vi "gatherdata_bakup2.vi"() -> ()   [LabVIEW 2011]
uses:
  <vilib>/FPGAPlugInAG/sbRIO-9606/niLvFpga_Open_sbRIO-9606.vi
  <vilib>/rvi/interface/common/dynamic/niFpgaDynamicAddResources.vi
  <vilib>/Utility/error.llb/Error Cluster From Error Code.vi
  <vilib>/rvi/errors/niLvFpgaAdjustHostInterfaceError.vi
  <vilib>/rvi/interface/nirviOpenFPGA/nirviOpenFPGA.xnode
  labview/FPGA Bitfiles/natcar_FPGATarget_Top-Level_610FB000.lvbitx
  <vilib>/rvi/interface/nirviReadWriteControl/nirviReadWriteControl.xnode
  NiFpgaLv.dll
  <vilib>/rvi/interface/Simulation/niFpgaSimulationCallBeginRW.vi
panel:
  in  "stop":bool
  in  "Save Path and Filename":path
  out "AI7":u16
  out "AI6":u16
  out "AI5":u16
  out "AI4":u16
  out "AI3":u16
  out "AI2":u16
  out "AI1":u16
  out "AI0":u16
  in  "#pts to avg":dbl=100000.0
  out "Waiting":bool
  out "Saving\nData":bool
  out "Getting\nData":bool
  in  "distance":dbl
  in  "Record":bool
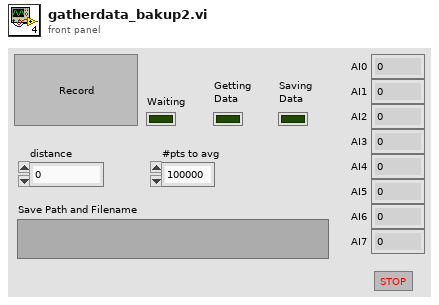
[diagram p1: front panel]
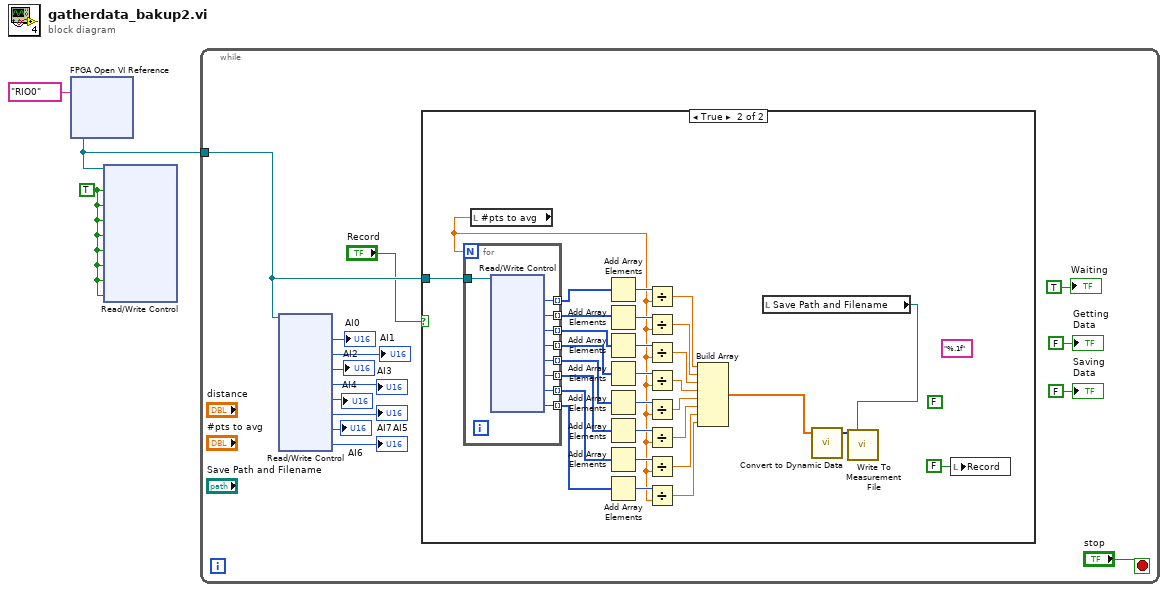
[diagram p0: block diagram]
diagram:
  w3 = TRUE ("Enable AI0")
  n1 = xnode "FPGA Open VI Reference"("resource name"=tag "RIO0") -> ("FPGA VI Reference Out"=w1:refnum<k20>)  [unwired: 1 in, 1 out]
  n2 = xnode "Read/Write Control"("FPGA VI Reference In"=w1, "Enable AI0"=w3, "Enable AI1"=w3, "Enable AI2"=w3, "Enable AI3"=w3, "Enable AI4"=w3, "Enable AI5"=w3, "Enable AI6"=w3, "Enable AI7"=w3) -> ()  [unwired: 1 in, 2 out]
  n3 = while {
    tunnel: w1 -> [w5]
    stop <- "stop" stop-if-true
    n4 = xnode "Read/Write Control"("FPGA VI Reference In"=w5) -> ("AI0"=→"AI0":u16, "AI1"=→"AI1":u16, "AI2"=→"AI2":u16, "AI3"=→"AI3":u16, "AI4"=→"AI4":u16, "AI5"=→"AI5":u16, "AI6"=→"AI6":u16, "AI7"=→"AI7":u16)  [unwired: 1 in, 2 out]
    n5 = case shown="True" "Record" {
      tunnel: w5 -> [_ w46]
      frame False {
      }
      frame True {
        (unwired) "%.1f" ("format (%.3f)")
        (unwired) FALSE ("append to file? (new file:F)")
        n6 = local read "#pts to avg"() -> (w29:dbl)
        n7 = for {
          N: w29 -> [_]
          tunnel: [w56] -> w38 mode=indexing
          tunnel: [w55] -> w37 mode=indexing
          tunnel: [w54] -> w36 mode=indexing
          tunnel: [w53] -> w34 mode=indexing
          tunnel: [w52] -> w35 mode=indexing
          tunnel: [w51] -> w33 mode=indexing
          tunnel: [w50] -> w32 mode=indexing
          tunnel: [w49] -> w30 mode=indexing
          tunnel: w46 -> [w48]
          n8 = xnode "Read/Write Control"("FPGA VI Reference In"=w48) -> ("AI0"=w56:u16, "AI1"=w55:u16, "AI2"=w54:u16, "AI3"=w52:u16, "AI4"=w53:u16, "AI5"=w51:u16, "AI6"=w50:u16, "AI7"=w49:u16)  [unwired: 1 in, 2 out]
        }
        n9 = Add Array Elements(numeric array=w38) -> (sum=w45:u16)
        n10 = Add Array Elements(numeric array=w37) -> (sum=w44:u16)
        n11 = Add Array Elements(numeric array=w36) -> (sum=w43:u16)
        n12 = Add Array Elements(numeric array=w35) -> (sum=w42:u16)
        n13 = Add Array Elements(numeric array=w34) -> (sum=w41:u16)
        n14 = Add Array Elements(numeric array=w33) -> (sum=w40:u16)
        n15 = Add Array Elements(numeric array=w32) -> (sum=w39:u16)
        n16 = Add Array Elements(numeric array=w30) -> (sum=w31:u16)
        n17 = Divide(x=w45, y=w29) -> (x/y=w28:dbl)
        n18 = Divide(x=w44, y=w29) -> (x/y=w27:dbl)
        n19 = Divide(x=w43, y=w29) -> (x/y=w26:dbl)
        n20 = Divide(x=w42, y=w29) -> (x/y=w25:dbl)
        n21 = Divide(x=w41, y=w29) -> (x/y=w21:dbl)
        n22 = Divide(x=w40, y=w29) -> (x/y=w22:dbl)
        n23 = Divide(x=w39, y=w29) -> (x/y=w23:dbl)
        n24 = Divide(x=w31, y=w29) -> (x/y=w24:dbl)
        n25 = Build Array(w28, w27, w26, w25, w21, w22, w23, w24) -> (w47:dbl[])
        n26 = local read "Save Path and Filename"() -> (w19:path)
        n27 = call "Convert to Dynamic Data"("Array"=w47) -> ("Dynamic Data Type"=w18:dynamicdata)  [unwired: 3 in]
        n28 = call "Write To Measurement File"("Signals"=w18, "Filename"=w19) -> ()  [unwired: 15 in, 3 out]
        n29 = local write "Record"(FALSE ("Record")) -> ()
      }
    }
    "Getting\nData" <- FALSE ("Getting\nData")
    "Saving\nData" <- FALSE ("Saving\nData")
    "Waiting" <- TRUE ("Waiting")
  }
